vi "SP Convert 5.0 to 5.1.vi"(0 "S Parameter 5.0 Test Parameters":T32={"Stimulus"={"Use Instrument Settings"=FALSE, "Blank Frequencies"=FALSE, "Sweep Type"=enum."Linear", "Sweep"={"Fstart"=0.0, "Fstop"=0.0, "Units"=enum."Hz", "Points"=2}, "Power (dBm)"=999.0, "IFBW (Hz)"=-1.0, "Sweep Time (s)"=-1.0, "Calibration"={"State"=FALSE, "String"=""}}, "Measurement"={"Auto Select"=FALSE, "Data Source"=enum."VNA", "Ports"=2, "Parameters"=[]}, "De-Embed"={"De-Embed"=FALSE, "Adapters"=[]}, "Display"={"Lock Control"=FALSE, "Retain Settings"=TRUE, "Formatted Data"=FALSE, "Plot Orientation"=enum."Single", "Plot Controls"=[{"Trace Orientation"=enum."Overlay", "Frequency"={"Change Frequency"=FALSE, "Start"=500.0, "Stop"=1500.0, "Units"=enum."MHz"}, "Markers"=[], "Traces"=[]}, {"Trace Orientation"=enum."Overlay", "Frequency"={"Change Frequency"=FALSE, "Start"=500.0, "Stop"=1500.0, "Units"=enum."MHz"}, "Markers"=[], "Traces"=[]}, {"Trace Orientation"=enum."Overlay", "Frequency"={"Change Frequency"=FALSE, "Start"=500.0, "Stop"=1500.0, "Units"=enum."MHz"}, "Markers"=[], "Traces"=[]}, {"Trace Orientation"=enum."Overlay", "Frequency"={"Change Frequency"=FALSE, "Start"=500.0, "Stop"=1500.0, "Units"=enum."MHz"}, "Markers"=[], "Traces"=[]}]}, "Limits"=[], "Filter Limits"=[]} {"Filter Limits"."Parameter"."Stimulus Port" min=1 step=1; "Filter Limits"."Parameter"."Response Port" min=1 step=1; "Filter Limits"."Passband"."Bandwidth Attn" format="%.3g"; "Filter Limits"."Passband"."Stop/Span" format="%.3g"; "Filter Limits"."Passband"."Start/Center" format="%.3g"; "Measurement"."Parameters"."Channel" min=0 max=32 step=1; "Measurement"."Parameters"."Parameter"."Stimulus Port" min=1 step=1; "Measurement"."Parameters"."Parameter"."Response Port" min=1 step=1; "Limits"."Parameter"."Stimulus Port" min=1 step=1; "Limits"."Parameter"."Response Port" min=1 step=1; "Stimulus"."Sweep Time (s)" format="%.3g"; "Display"."Plot Controls"."Traces"."Reference" format="%#.2g"; "Display"."Plot Controls"."Traces"."Display Data" items=["Data", "Memory", "Data/Memory"]; "Display"."Plot Controls"."Traces"."Format" items=["Log Mag", "Phase", "Expanded Phase", "Delay", "Smith", "Polar", "Lin Mag", "SWR", "Loss", "Real", "Imaginary"]; "Display"."Plot Controls"."Traces"."Scale" min=0.001 step=1.0 format="%#.2g"; "Display"."Plot Controls"."Traces"."Position" min=0.0 max=10.0; "Display"."Plot Controls"."Frequency"."Stop" format="%.3g"; "Display"."Plot Controls"."Frequency"."Start" format="%.3g"}) -> (2 "S Parameter 5.1 Test Parameters":T1={"Stimulus"={"Use Instrument Settings"=FALSE, "Blank Frequencies"=FALSE, "Sweep Type"=enum."Linear", "Sweep"={"Fstart"=500.0, "Fstop"=1500.0, "Units"=enum."MHz", "Points"=2}, "Power (dBm)"=999.0, "IFBW (Hz)"=-1.0, "Sweep Time (s)"=-1.0, "Calibration"={"State"=FALSE, "String"=""}}, "Measurement"={"Auto Select"=TRUE, "Data Source"=enum."VNA", "Ports"=2, "Parameters"=[]}, "De-Embed"={"De-Embed"=FALSE, "Adapters"=[]}, "Display"={"Lock Control"=FALSE, "Retain Settings"=TRUE, "Formatted Data"=FALSE, "Plot Orientation"=enum."Single", "Plot Controls"=[{"Trace Orientation"=enum."Overlay", "Frequency"={"Change Frequency"=FALSE, "Start"=500.0, "Stop"=1500.0, "Units"=enum."MHz"}, "Markers"=[], "Traces"=[]}, {"Trace Orientation"=enum."Overlay", "Frequency"={"Change Frequency"=FALSE, "Start"=500.0, "Stop"=1500.0, "Units"=enum."MHz"}, "Markers"=[], "Traces"=[]}, {"Trace Orientation"=enum."Overlay", "Frequency"={"Change Frequency"=FALSE, "Start"=500.0, "Stop"=1500.0, "Units"=enum."MHz"}, "Markers"=[], "Traces"=[]}, {"Trace Orientation"=enum."Overlay", "Frequency"={"Change Frequency"=FALSE, "Start"=500.0, "Stop"=1500.0, "Units"=enum."MHz"}, "Markers"=[], "Traces"=[]}]}, "Limits"=[], "Filter Limits"=[]} {"Filter Limits"."Parameter"."Stimulus Port" min=1 step=1; "Filter Limits"."Parameter"."Response Port" min=1 step=1; "Filter Limits"."Passband"."Bandwidth Attn" format="%.3g"; "Filter Limits"."Passband"."Stop/Span" format="%.3g"; "Filter Limits"."Passband"."Start/Center" format="%.3g"; "Measurement"."Parameters"."Channel" min=0 max=32 step=1; "Measurement"."Parameters"."Parameter"."Stimulus Port" min=1 step=1; "Measurement"."Parameters"."Parameter"."Response Port" min=1 step=1; "Limits"."Parameter"."Stimulus Port" min=1 step=1; "Limits"."Parameter"."Response Port" min=1 step=1; "Stimulus"."Sweep Time (s)" format="%.3g"; "Display"."Plot Controls"."Traces"."Reference" format="%#.2g"; "Display"."Plot Controls"."Traces"."Display Data" items=["Data", "Memory", "Data/Memory"]; "Display"."Plot Controls"."Traces"."Format" items=["Log Mag", "Phase", "Expanded Phase", "Delay", "Smith", "Polar", "Lin Mag", "SWR", "Loss", "Real", "Imaginary"]; "Display"."Plot Controls"."Traces"."Scale" min=0.001 step=1.0 format="%#.2g"; "Display"."Plot Controls"."Traces"."Position" min=0.0 max=10.0; "Display"."Plot Controls"."Frequency"."Stop" format="%.3g"; "Display"."Plot Controls"."Frequency"."Start" format="%.3g"})   [LabVIEW 2011]
uses:
  TypeDefs/SP Test Parameters v5.0.ctl
  TypeDefs/SP Test Parameters.ctl
  TypeDefs/SP Stimulus Parameters.ctl
  TypeDefs/SP Frequency Units.ctl
  TypeDefs/SP Calibration State.ctl
  TypeDefs/SP Measurement.ctl
  TypeDefs/SP Parameters.ctl
  TypeDefs/SP Parameter.ctl
  TypeDefs/SP De-Embed.ctl
  TypeDefs/SP Adapter.ctl
  TypeDefs/SP Data.ctl
  TypeDefs/SP Display Parameters.ctl
  TypeDefs/SP Display Plot Controls Cluster.ctl
  TypeDefs/SP Marker Cluster.ctl
  TypeDefs/SP Marker Type.ctl
  TypeDefs/SP Display Trace Controls.ctl
  TypeDefs/SP Display Format.ctl
  TypeDefs/SP Display Data.ctl
  TypeDefs/SP Limit.ctl
  TypeDefs/SP Format.ctl
  TypeDefs/SP Limit Type.ctl
  TypeDefs/SP Limit Point.ctl
  Test Referential Limit.ctl
  TypeDefs/SP Filter.ctl
  TypeDefs/SP Filter Type.ctl
  TypeDefs/SP Filter Passband.ctl
  TypeDefs/SP Frequency Format.ctl
  TypeDefs/SP Filter Ripple.ctl
  TypeDefs/SP Attenuation Point.ctl
  TypeDefs/SP Attenuation Type.ctl
  TypeDefs/SP Skirt Rejection Point.ctl
  TypeDefs/SP Relative Loss.ctl
panel:
  # "Div"
  # "Div"
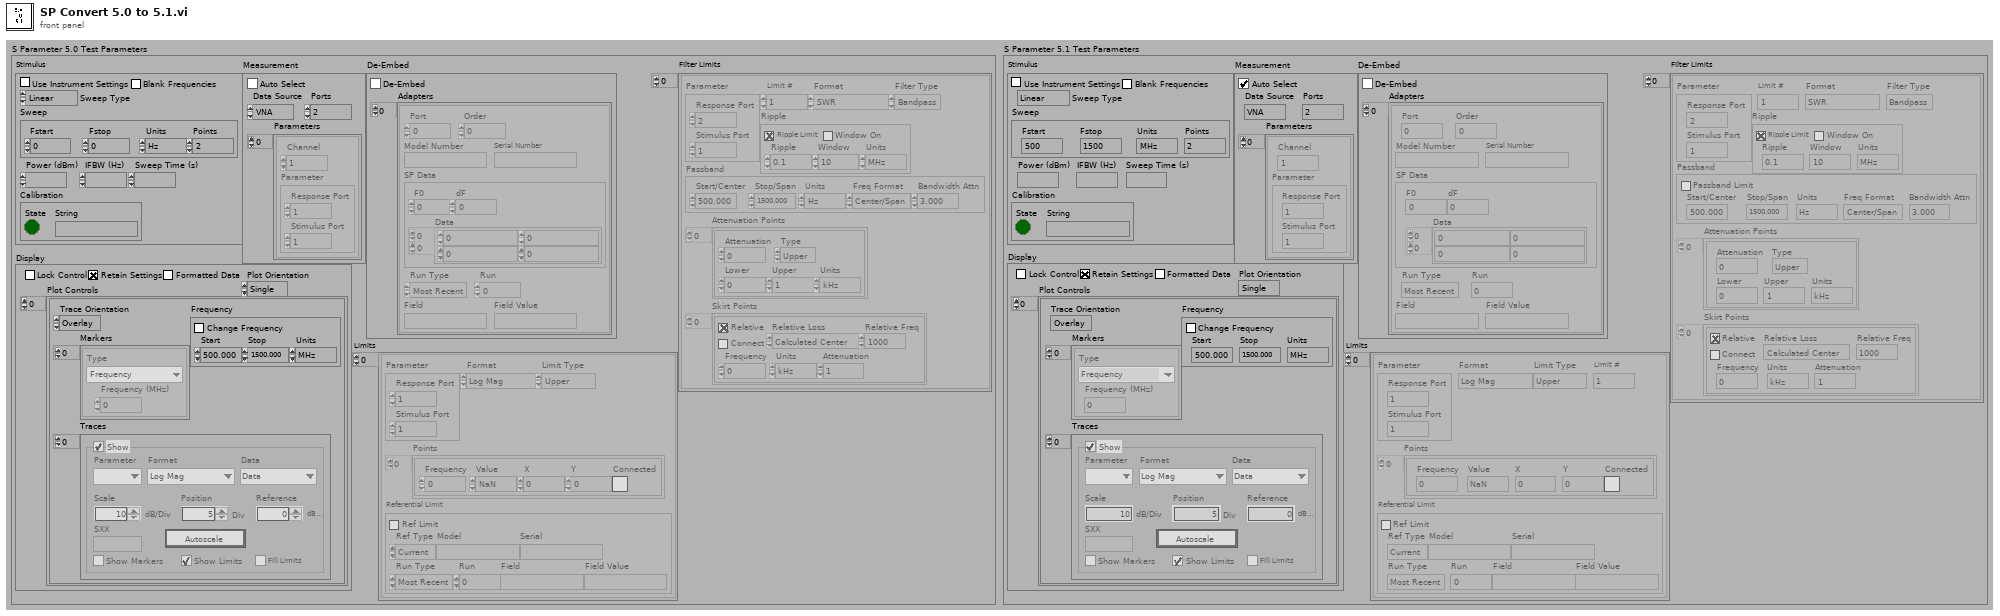
[diagram p1: front panel]
types:
  T1 = typedef "SP Test Parameters.ctl" = cluster{"Stimulus":T2, "Measurement":T5, "De-Embed":T8, "Display":T11, "Limits":T18[], "Filter Limits":T23[]}
  T2 = typedef "SP Stimulus Parameters.ctl" = cluster{"Use Instrument Settings":bool, "Blank Frequencies":bool, "Sweep Type":enum32{"Linear", "Logarithmic", "List", "Power", "CW"}, "Sweep":cluster{"Fstart":dbl, "Fstop":dbl, "Units":T3, "Points":i32}, "Power (dBm)":dbl, "IFBW (Hz)":dbl, "Sweep Time (s)":dbl, "Calibration":T4}
  T3 = typedef "SP Frequency Units.ctl" = enum16{"Hz", "kHz", "MHz", "GHz", "Points"}
  T4 = typedef "SP Calibration State.ctl" = cluster{"State":bool, "String":string}
  T5 = typedef "SP Measurement.ctl" = cluster{"Auto Select":bool, "Data Source":enum16{"VNA", "Data File"}, "Ports":i8, "Parameters":T6[]}
  T6 = typedef "SP Parameters.ctl" = cluster{"Channel":i8, "Parameter":T7}
  T7 = typedef "SP Parameter.ctl" = cluster{"Stimulus Port":i8, "Response Port":i8}
  T8 = typedef "SP De-Embed.ctl" = cluster{"De-Embed":bool, "Adapters":T9[]}
  T9 = typedef "SP Adapter.ctl" = cluster{"Port":i8, "Order":i8, "Model Number":string, "Serial Number":string, "SP Data":T10, "Run Type":enum16{"Most Recent", "Run #", "Match Field"}, "Run":i32, "Field":string, "Field Value":string}
  T10 = typedef "SP Data.ctl" = cluster{"F0":dbl, "dF":dbl, "Data":cdb[][]}
  T11 = typedef "SP Display Parameters.ctl" = cluster{"Lock Control":bool, "Retain Settings":bool, "Formatted Data":bool, "Plot Orientation":enum32{"Single", "Dual", "Quad"}, "Plot Controls":T12[]}
  T12 = typedef "SP Display Plot Controls Cluster.ctl" = cluster{"Trace Orientation":enum32{"Overlay", "Split"}, "Frequency":cluster{"Change Frequency":bool, "Start":dbl, "Stop":dbl, "Units":T3}, "Markers":T13[], "Traces":T15[]}
  T13 = typedef "SP Marker Cluster.ctl" = cluster{"Type":T14, "Frequency (MHz)":dbl}
  T14 = typedef "SP Marker Type.ctl" = enum16{"Frequency", "Trace Maximum", "Trace Minimum", "Limit Maximum", "Limit Minimum"}
  T15 = typedef "SP Display Trace Controls.ctl" = cluster{"Trace On":bool, "Measure":i32, "Format":T16, "Autoscale":bool, "Reference":dbl, "\nRefUnit":string, "Position":dbl, "Scale":dbl, "ScaleUnit":string, "LimitOn":bool, "LimitFill":bool, "Display Data":T17, "Show Markers":bool, "SXX":string}
  T16 = typedef "SP Display Format.ctl" = i32
  T17 = typedef "SP Display Data.ctl" = u16
  T18 = typedef "SP Limit.ctl" = cluster{"Parameter":T7, "Format":T19, "Limit Type":T20, "Points":T21[], "Referential Limit":T22, "Limit #":i8}
  T19 = typedef "SP Format.ctl" = enum16{"Log Mag", "Lin Mag", "SWR", "Phase", "Expanded Phase", "Delay", "Insertion Loss", "Isolation", "Return Loss"}
  T20 = typedef "SP Limit Type.ctl" = enum16{"Upper", "Lower", "Delta", "Filter", "Referential"}
  T21 = typedef "SP Limit Point.ctl" = cluster{"Frequency":dbl, "Value":dbl, "X":dbl, "Y":dbl, "Connected":bool}
  T22 = typedef "Test Referential Limit.ctl" = cluster{"Ref Limit":bool, "Ref Type":enum16{"Current", "Specify"}, "Model":string, "Serial":string, "Run Type":enum16{"Most Recent", "Run #", "Match Field"}, "Run":i32, "Field":string, "Field Value":string}
  T23 = typedef "SP Filter.ctl" = cluster{"Limit #":i8, "Parameter":T7, "Format":T19, "Filter Type":T24, "Passband":T25, "Ripple":T27, "Attenuation Points":T28[], "Skirt Points":T30[]}
  T24 = typedef "SP Filter Type.ctl" = enum16{"Lowpass", "Highpass", "Bandpass", "Bandstop"}
  T25 = typedef "SP Filter Passband.ctl" = cluster{"Start/Center":dbl, "Stop/Span":dbl, "Units":T3, "Freq Format":T26, "Bandwidth Attn":dbl, "Passband Limit":bool}
  T26 = typedef "SP Frequency Format.ctl" = enum16{"Start/Stop", "Center/Span"}
  T27 = typedef "SP Filter Ripple.ctl" = cluster{"Ripple Limit":bool, "Window On":bool, "Ripple":dbl, "Window":dbl, "Units":T3}
  T28 = typedef "SP Attenuation Point.ctl" = cluster{"Attenuation":dbl, "Type":T29, "Lower":dbl, "Upper":dbl, "Units":T3}
  T29 = typedef "SP Attenuation Type.ctl" = enum16{"Center", "Lower", "Upper"}
  T30 = typedef "SP Skirt Rejection Point.ctl" = cluster{"Relative":bool, "Connect":bool, "Frequency":dbl, "Units":T3, "Attenuation":dbl, "Relative Loss":T31, "Relative Freq":dbl}
  T31 = typedef "SP Relative Loss.ctl" = enum16{"Calculated Center", "Passband Minimum", "Passband Maximum", "Passband Average", "Frequency"}
  T32 = typedef "SP Test Parameters v5.0.ctl" = cluster{"Stimulus":cluster{"Use Instrument Settings":bool, "Blank Frequencies":bool, "Sweep Type":enum32{"Linear", "Logarithmic", "List", "Power", "CW"}, "Sweep":cluster{"Fstart":dbl, "Fstop":dbl, "Units":enum16{"Hz", "kHz", "MHz", "GHz", "Points"}, "Points":i32}, "Power (dBm)":dbl, "IFBW (Hz)":dbl, "Sweep Time (s)":dbl, "Calibration":cluster{"State":bool, "String":string}}, "Measurement":cluster{"Auto Select":bool, "Data Source":enum16{"VNA", "Data File"}, "Ports":i8, "Parameters":cluster{"Channel":i8, "Parameter":cluster{"Stimulus Port":i8, "Response Port":i8}}[]}, "De-Embed":cluster{"De-Embed":bool, "Adapters":cluster{"Port":i8, "Order":i8, "Model Number":string, "Serial Number":string, "SP Data":cluster{"F0":dbl, "dF":dbl, "Data":cdb[][]}, "Run Type":enum16{"Most Recent", "Run #", "Match Field"}, "Run":i32, "Field":string, "Field Value":string}[]}, "Display":cluster{"Lock Control":bool, "Retain Settings":bool, "Formatted Data":bool, "Plot Orientation":enum32{"Single", "Dual", "Quad"}, "Plot Controls":cluster{"Trace Orientation":enum32{"Overlay", "Split"}, "Frequency":cluster{"Change Frequency":bool, "Start":dbl, "Stop":dbl, "Units":enum16{"Hz", "kHz", "MHz", "GHz", "Points"}}, "Markers":cluster{"Type":enum16{"Frequency", "Trace Maximum", "Trace Minimum", "Limit Maximum", "Limit Minimum"}, "Frequency (MHz)":dbl}[], "Traces":cluster{"Trace On":bool, "Measure":i32, "Format":i32, "Autoscale":bool, "Reference":dbl, "\nRefUnit":string, "Position":dbl, "Scale":dbl, "ScaleUnit":string, "LimitOn":bool, "LimitFill":bool, "Display Data":u16, "Show Markers":bool, "SXX":string}[]}[]}, "Limits":cluster{"Parameter":cluster{"Stimulus Port":i8, "Response Port":i8}, "Format":enum16{"Log Mag", "Lin Mag", "SWR", "Phase", "Expanded Phase", "Delay", "Insertion Loss", "Isolation", "Return Loss"}, "Limit Type":enum16{"Upper", "Lower", "Delta", "Filter", "Referential"}, "Points":cluster{"Frequency":dbl, "Value":dbl, "X":dbl, "Y":dbl, "Connected":bool}[], "Referential Limit":cluster{"Ref Limit":bool, "Ref Type":enum16{"Current", "Specify"}, "Model":string, "Serial":string, "Run Type":enum16{"Most Recent", "Run #", "Match Field"}, "Run":i32, "Field":string, "Field Value":string}}[], "Filter Limits":cluster{"Limit #":i8, "Parameter":cluster{"Stimulus Port":i8, "Response Port":i8}, "Format":enum16{"Log Mag", "Lin Mag", "SWR", "Phase", "Expanded Phase", "Delay", "Insertion Loss", "Isolation", "Return Loss"}, "Filter Type":enum16{"Lowpass", "Highpass", "Bandpass", "Bandstop"}, "Passband":cluster{"Start/Center":dbl, "Stop/Span":dbl, "Units":enum16{"Hz", "kHz", "MHz", "GHz", "Points"}, "Freq Format":enum16{"Start/Stop", "Center/Span"}, "Bandwidth Attn":dbl}, "Ripple":cluster{"Ripple Limit":bool, "Window On":bool, "Ripple":dbl, "Window":dbl, "Units":enum16{"Hz", "kHz", "MHz", "GHz", "Points"}}, "Attenuation Points":cluster{"Attenuation":dbl, "Type":enum16{"Center", "Lower", "Upper"}, "Lower":dbl, "Upper":dbl, "Units":enum16{"Hz", "kHz", "MHz", "GHz", "Points"}}[], "Skirt Points":cluster{"Relative":bool, "Connect":bool, "Frequency":dbl, "Units":enum16{"Hz", "kHz", "MHz", "GHz", "Points"}, "Attenuation":dbl, "Relative Loss":enum16{"Calculated Center", "Passband Minimum", "Passband Maximum", "Passband Average", "Frequency"}, "Relative Freq":dbl}[]}[]}
  T33 = cluster{"Use Instrument Settings":bool, "Blank Frequencies":bool, "Sweep Type":enum32{"Linear", "Logarithmic", "List", "Power", "CW"}, "Sweep":cluster{"Fstart":dbl, "Fstop":dbl, "Units":enum16{"Hz", "kHz", "MHz", "GHz", "Points"}, "Points":i32}, "Power (dBm)":dbl, "IFBW (Hz)":dbl, "Sweep Time (s)":dbl, "Calibration":cluster{"State":bool, "String":string}}
  T34 = cluster{"Auto Select":bool, "Data Source":enum16{"VNA", "Data File"}, "Ports":i8, "Parameters":cluster{"Channel":i8, "Parameter":cluster{"Stimulus Port":i8, "Response Port":i8}}[]}
  T35 = cluster{"De-Embed":bool, "Adapters":cluster{"Port":i8, "Order":i8, "Model Number":string, "Serial Number":string, "SP Data":cluster{"F0":dbl, "dF":dbl, "Data":cdb[][]}, "Run Type":enum16{"Most Recent", "Run #", "Match Field"}, "Run":i32, "Field":string, "Field Value":string}[]}
  T36 = cluster{"Lock Control":bool, "Retain Settings":bool, "Formatted Data":bool, "Plot Orientation":enum32{"Single", "Dual", "Quad"}, "Plot Controls":cluster{"Trace Orientation":enum32{"Overlay", "Split"}, "Frequency":cluster{"Change Frequency":bool, "Start":dbl, "Stop":dbl, "Units":enum16{"Hz", "kHz", "MHz", "GHz", "Points"}}, "Markers":cluster{"Type":enum16{"Frequency", "Trace Maximum", "Trace Minimum", "Limit Maximum", "Limit Minimum"}, "Frequency (MHz)":dbl}[], "Traces":cluster{"Trace On":bool, "Measure":i32, "Format":i32, "Autoscale":bool, "Reference":dbl, "\nRefUnit":string, "Position":dbl, "Scale":dbl, "ScaleUnit":string, "LimitOn":bool, "LimitFill":bool, "Display Data":u16, "Show Markers":bool, "SXX":string}[]}[]}
  T37 = cluster{"Parameter":cluster{"Stimulus Port":i8, "Response Port":i8}, "Format":enum16{"Log Mag", "Lin Mag", "SWR", "Phase", "Expanded Phase", "Delay", "Insertion Loss", "Isolation", "Return Loss"}, "Limit Type":enum16{"Upper", "Lower", "Delta", "Filter", "Referential"}, "Points":cluster{"Frequency":dbl, "Value":dbl, "X":dbl, "Y":dbl, "Connected":bool}[], "Referential Limit":cluster{"Ref Limit":bool, "Ref Type":enum16{"Current", "Specify"}, "Model":string, "Serial":string, "Run Type":enum16{"Most Recent", "Run #", "Match Field"}, "Run":i32, "Field":string, "Field Value":string}}[]
  T38 = cluster{"Limit #":i8, "Parameter":cluster{"Stimulus Port":i8, "Response Port":i8}, "Format":enum16{"Log Mag", "Lin Mag", "SWR", "Phase", "Expanded Phase", "Delay", "Insertion Loss", "Isolation", "Return Loss"}, "Filter Type":enum16{"Lowpass", "Highpass", "Bandpass", "Bandstop"}, "Passband":cluster{"Start/Center":dbl, "Stop/Span":dbl, "Units":enum16{"Hz", "kHz", "MHz", "GHz", "Points"}, "Freq Format":enum16{"Start/Stop", "Center/Span"}, "Bandwidth Attn":dbl}, "Ripple":cluster{"Ripple Limit":bool, "Window On":bool, "Ripple":dbl, "Window":dbl, "Units":enum16{"Hz", "kHz", "MHz", "GHz", "Points"}}, "Attenuation Points":cluster{"Attenuation":dbl, "Type":enum16{"Center", "Lower", "Upper"}, "Lower":dbl, "Upper":dbl, "Units":enum16{"Hz", "kHz", "MHz", "GHz", "Points"}}[], "Skirt Points":cluster{"Relative":bool, "Connect":bool, "Frequency":dbl, "Units":enum16{"Hz", "kHz", "MHz", "GHz", "Points"}, "Attenuation":dbl, "Relative Loss":enum16{"Calculated Center", "Passband Minimum", "Passband Maximum", "Passband Average", "Frequency"}, "Relative Freq":dbl}[]}[]
  T39 = enum16{"Log Mag", "Lin Mag", "SWR", "Phase", "Expanded Phase", "Delay", "Insertion Loss", "Isolation", "Return Loss"}
  T40 = enum16{"Upper", "Lower", "Delta", "Filter", "Referential"}
  T41 = cluster{"Frequency":dbl, "Value":dbl, "X":dbl, "Y":dbl, "Connected":bool}[]
  T42 = cluster{"Ref Limit":bool, "Ref Type":enum16{"Current", "Specify"}, "Model":string, "Serial":string, "Run Type":enum16{"Most Recent", "Run #", "Match Field"}, "Run":i32, "Field":string, "Field Value":string}
  T43 = enum16{"Lowpass", "Highpass", "Bandpass", "Bandstop"}
  T44 = cluster{"Ripple Limit":bool, "Window On":bool, "Ripple":dbl, "Window":dbl, "Units":enum16{"Hz", "kHz", "MHz", "GHz", "Points"}}
  T45 = cluster{"Attenuation":dbl, "Type":enum16{"Center", "Lower", "Upper"}, "Lower":dbl, "Upper":dbl, "Units":enum16{"Hz", "kHz", "MHz", "GHz", "Points"}}[]
  T46 = cluster{"Relative":bool, "Connect":bool, "Frequency":dbl, "Units":enum16{"Hz", "kHz", "MHz", "GHz", "Points"}, "Attenuation":dbl, "Relative Loss":enum16{"Calculated Center", "Passband Minimum", "Passband Maximum", "Passband Average", "Frequency"}, "Relative Freq":dbl}[]
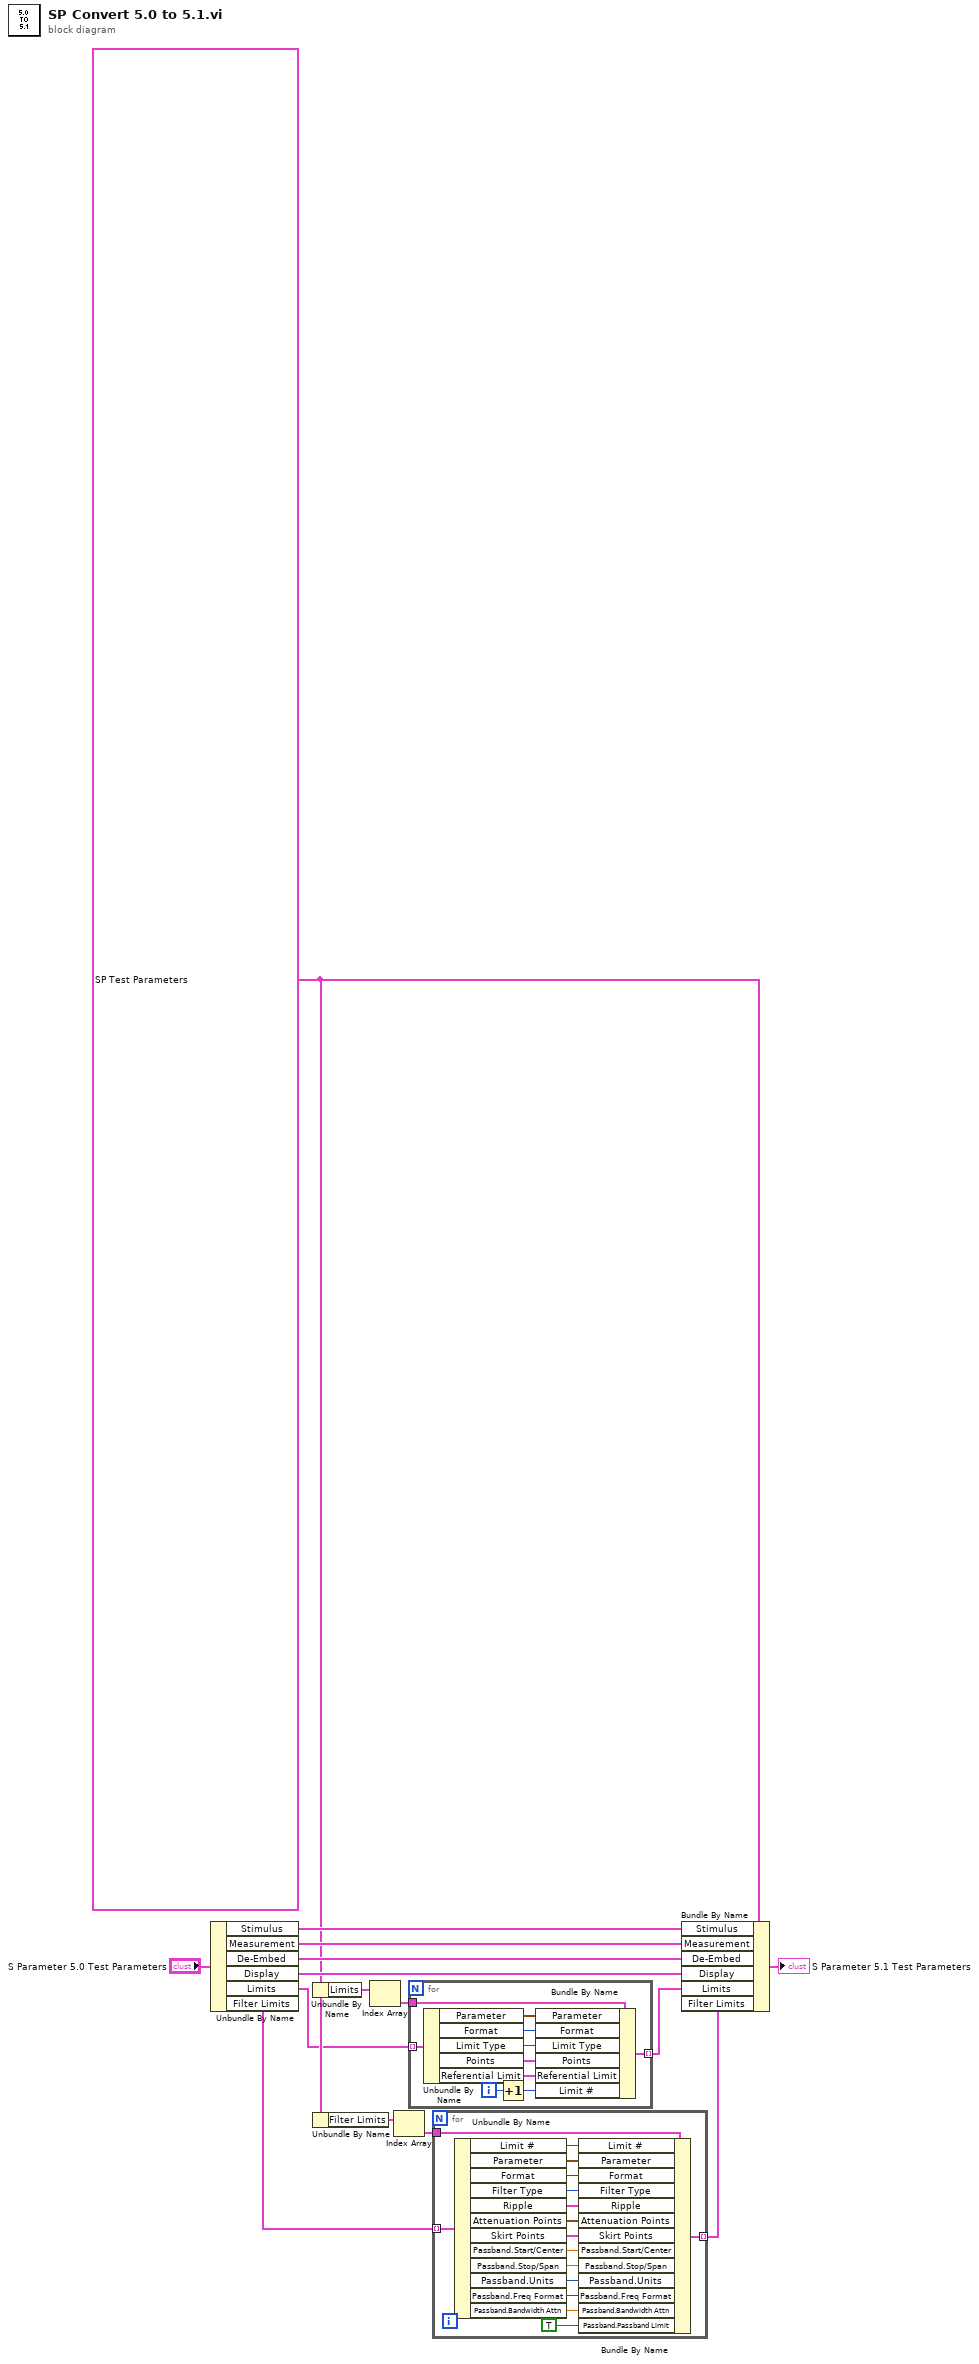
[diagram p0: block diagram]
diagram:
  w3 = T1 {"Stimulus"={"Use Instrument Settings"=FALSE, "Blank Frequencies"=FALSE, "Sweep Type"=enum."Linear", "Sweep"={"Fstart"=0.0, "Fstop"=0.0, "Units"=enum."Hz", "Points"=0}, "Power (dBm)"=0.0, "IFBW (Hz)"=0.0, "Sweep Time (s)"=0.0, "Calibration"={"State"=FALSE, "String"=""}}, "Measurement"={"Auto Select"=FALSE, "Data Source"=enum."VNA", "Ports"=0, "Parameters"=[]}, "De-Embed"={"De-Embed"=FALSE, "Adapters"=[]}, "Display"={"Lock Control"=FALSE, "Retain Settings"=FALSE, "Formatted Data"=FALSE, "Plot Orientation"=enum."Single", "Plot Controls"=[{"Trace Orientation"=enum."Overlay", "Frequency"={"Change Frequency"=FALSE, "Start"=0.0, "Stop"=0.0, "Units"=enum."Hz"}, "Markers"=[], "Traces"=[{"Trace On"=TRUE, "Measure"=0, "Format"=0, "Autoscale"=TRUE, "Reference"=0.0, "\nRefUnit"="dB/Div", "Position"=5.0, "Scale"=10.0, "ScaleUnit"="dB/Div", "LimitOn"=TRUE, "LimitFill"=FALSE, "Display Data"=0, "Show Markers"=FALSE, "SXX"="S11"}, {"Trace On"=TRUE, "Measure"=0, "Format"=0, "Autoscale"=TRUE, "Reference"=0.0, "\nRefUnit"="dB/Div", "Position"=5.0, "Scale"=10.0, "ScaleUnit"="dB/Div", "LimitOn"=TRUE, "LimitFill"=FALSE, "Display Data"=0, "Show Markers"=FALSE, "SXX"="S21"}]}, {"Trace Orientation"=enum."Overlay", "Frequency"={"Change Frequency"=FALSE, "Start"=0.0, "Stop"=0.0, "Units"=enum."Hz"}, "Markers"=[], "Traces"=[{"Trace On"=TRUE, "Measure"=0, "Format"=0, "Autoscale"=TRUE, "Reference"=0.0, "\nRefUnit"="dB/Div", "Position"=5.0, "Scale"=10.0, "ScaleUnit"="dB/Div", "LimitOn"=TRUE, "LimitFill"=FALSE, "Display Data"=0, "Show Markers"=FALSE, "SXX"="S11"}, {"Trace On"=TRUE, "Measure"=0, "Format"=0, "Autoscale"=TRUE, "Reference"=0.0, "\nRefUnit"="dB/Div", "Position"=5.0, "Scale"=10.0, "ScaleUnit"="dB/Div", "LimitOn"=TRUE, "LimitFill"=FALSE, "Display Data"=0, "Show Markers"=FALSE, "SXX"="S21"}]}, {"Trace Orientation"=enum."Overlay", "Frequency"={"Change Frequency"=FALSE, "Start"=0.0, "Stop"=0.0, "Units"=enum."Hz"}, "Markers"=[], "Traces"=[{"Trace On"=TRUE, "Measure"=0, "Format"=0, "Autoscale"=TRUE, "Reference"=0.0, "\nRefUnit"="dB/Div", "Position"=5.0, "Scale"=10.0, "ScaleUnit"="dB/Div", "LimitOn"=TRUE, "LimitFill"=FALSE, "Display Data"=0, "Show Markers"=FALSE, "SXX"="S11"}, {"Trace On"=TRUE, "Measure"=0, "Format"=0, "Autoscale"=TRUE, "Reference"=0.0, "\nRefUnit"="dB/Div", "Position"=5.0, "Scale"=10.0, "ScaleUnit"="dB/Div", "LimitOn"=TRUE, "LimitFill"=FALSE, "Display Data"=0, "Show Markers"=FALSE, "SXX"="S21"}]}, {"Trace Orientation"=enum."Overlay", "Frequency"={"Change Frequency"=FALSE, "Start"=0.0, "Stop"=0.0, "Units"=enum."Hz"}, "Markers"=[], "Traces"=[{"Trace On"=TRUE, "Measure"=0, "Format"=0, "Autoscale"=TRUE, "Reference"=0.0, "\nRefUnit"="dB/Div", "Position"=5.0, "Scale"=10.0, "ScaleUnit"="dB/Div", "LimitOn"=TRUE, "LimitFill"=FALSE, "Display Data"=0, "Show Markers"=FALSE, "SXX"="S11"}, {"Trace On"=TRUE, "Measure"=0, "Format"=0, "Autoscale"=TRUE, "Reference"=0.0, "\nRefUnit"="dB/Div", "Position"=5.0, "Scale"=10.0, "ScaleUnit"="dB/Div", "LimitOn"=TRUE, "LimitFill"=FALSE, "Display Data"=0, "Show Markers"=FALSE, "SXX"="S21"}]}]}, "Limits"=[], "Filter Limits"=[]} ("S Parameter Test Parameters")
  n1 = Unbundle By Name("S Parameter 5.0 Test Parameters") -> ("Stimulus"=w11:T33, "Measurement"=w8:T34, "De-Embed"=w9:T35, "Display"=w10:T36, "Limits"=w2:T37, "Filter Limits"=w7:T38)
  n2 = Unbundle By Name(w3) -> ("Limits"=w4:T18[])
  n3 = Unbundle By Name(w3) -> ("Filter Limits"=w13:T23[])
  n4 = Index Array(array=w4) -> (element=w5:T18)  [unwired: 1 in]
  n5 = Index Array(array=w13) -> (element=w12:T23)  [unwired: 1 in]
  n6 = for {
    tunnel: w2 -> [w25] mode=indexing
    tunnel: w5 -> [w21]
    tunnel: [w24] -> w1 mode=indexing
    i -> [w17]
    n7 = Unbundle By Name(w25) -> ("Parameter"=w23:cluster{"Stimulus Port":i8, "Response Port":i8}, "Format"=w22:T39, "Limit Type"=w19:T40, "Points"=w20:T41, "Referential Limit"=w18:T42)
    n8 = Increment(x=w17) -> (x+1=w16:i32)
    n9 = Bundle By Name(cluster=w21, "Parameter"=w23, "Format"=w22, "Limit Type"=w19, "Points"=w20, "Referential Limit"=w18, "Limit #"=w16) -> (w24:T18)
  }
  n10 = for {
    tunnel: w7 -> [w41] mode=indexing
    tunnel: w12 -> [w37]
    tunnel: [w40] -> w6 mode=indexing
    n11 = Unbundle By Name(w41) -> ("Limit #"=w39:i8, "Parameter"=w38:cluster{"Stimulus Port":i8, "Response Port":i8}, "Format"=w33:T39, "Filter Type"=w34:T43, "Ripple"=w32:T44, "Attenuation Points"=w35:T45, "Skirt Points"=w36:T46, "Passband.Start/Center"=w27:dbl, "Passband.Stop/Span"=w28:dbl, "Passband.Units"=w29:enum16{"Hz", "kHz", "MHz", "GHz", "Points"}, "Passband.Freq Format"=w30:enum16{"Start/Stop", "Center/Span"}, "Passband.Bandwidth Attn"=w31:dbl)
    n12 = Bundle By Name(cluster=w37, "Limit #"=w39, "Parameter"=w38, "Format"=w33, "Filter Type"=w34, "Ripple"=w32, "Attenuation Points"=w35, "Skirt Points"=w36, "Passband.Start/Center"=w27, "Passband.Stop/Span"=w28, "Passband.Units"=w29, "Passband.Freq Format"=w30, "Passband.Bandwidth Attn"=w31, "Passband.Passband Limit"=TRUE) -> (w40:T23)
  }
  n13 = Bundle By Name(cluster=w3, "Stimulus"=w11, "Measurement"=w8, "De-Embed"=w9, "Display"=w10, "Limits"=w1, "Filter Limits"=w6) -> (→"S Parameter 5.1 Test Parameters":T1)
